vi "sq_test_all.vi"() -> ()   [LabVIEW 2012]
doc: "This VI is an example of how to use the Host VI to open the I2C bus, write, read, and close I2C bus. This VI should work for any I2C EEPROM or RAM IC. Note that many of these devices have a limit on how many bytes can be writen to the device at a time.\n\nWritten By:\nPeter Fuller\nSenior Engineer\nplf Consulting, LLC\n\nemail: peter@plfconsulting.com\nphone: 617.699.2201"
uses:
  <vilib>/Platform/TimedLoop/XDataNode/timing_clust.ctl
  <vilib>/Platform/TimedLoop/XDataNode/nitl_modes.ctl
  <vilib>/Platform/TimedLoop/XDataNode/wakeup.ctl
  <vilib>/Platform/TimedLoop/XDataNode/XDataNode.xnode
  <vilib>/Platform/TimedLoop/XDataNode/XDNodeRunTimeDep.lvlib
panel:
  in  "Send":bool
  in  "Bit rate":dbl=400000.0 min=40000.0 max=2000000.0 format="%#_3p"
  in  "Init sequences":T1={"Cluster"={"Cmd bytes"=[0, 99, 145], "Send"=FALSE}, "Cluster 2"={"Cmd bytes"=[0, 107, 145, 119, 255], "Send"=FALSE}, "Cluster 3"={"Cmd bytes"=[0, 103, 145, 119, 255], "Send"=FALSE}} {"Cluster 3"."Cmd bytes" format="%.0x"; "Cluster 2"."Cmd bytes" format="%.0x"; "Cluster"."Cmd bytes" format="%.0x"}
  in  "Cont":bool
  out "Run":bool
  in  "Steps":i32=10
  in  "Pulse count":cluster{"Pulse count 2":i16, "Array":bool[]}[](array[cluster])=[{"Pulse count 2"=0, "Array"=[FALSE, FALSE, FALSE, FALSE, FALSE, FALSE]}, {"Pulse count 2"=0, "Array"=[FALSE, FALSE, FALSE, FALSE, FALSE, FALSE]}, {"Pulse count 2"=0, "Array"=[FALSE, FALSE, FALSE, FALSE, FALSE, FALSE]}] {"Pulse count 2" min=-2047 max=2047 scale=-100.0..100.0}
  in  "Step":bool
  in  "Stop":bool
  # "Start address"
  # "First data byte"
  # "No-cal"
  # "Sweep"
  # "Incremental"
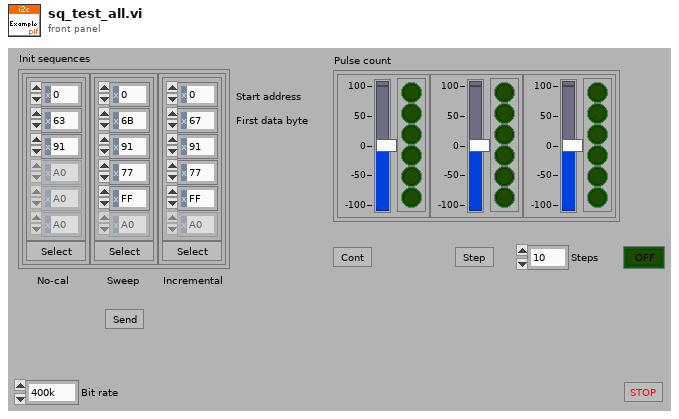
[diagram p1: front panel]
types:
  T1 = cluster{"Cluster":cluster{"Cmd bytes":u8[], "Send":bool}, "Cluster 2":cluster{"Cmd bytes":u8[], "Send":bool}, "Cluster 3":cluster{"Cmd bytes":u8[], "Send":bool}}
  T2 = typedef "i2c_interface.ctl" = cluster{"FPGA VI Reference":T3}
  T3 = typedef "fpga_reference.ctl" = refnum<k20>
  T4 = typedef "XDNodeRunTimeDep.lvlib/timing_clust.ctl" = cluster{"Expected End [f-1]":u64, "Actual End [f-1]":u64, "Finished Late? [f-1]":bool, "Expected End [i-1]":u64, "Actual End [i-1]":u64, "Finished Late? [i-1]":bool, "Expected Start [i]":u64, "Actual Start [i]":u64, "Expected Start [f]":u64, "Actual Start [f]":u64, "Source Name":string, "Structure Name":string, "Period":i64, "Deadline":i64, "Offset":i64, "Start":i64, "Priority":i32, "Timeout":i32, "Mode":T5, "Wakeup Reason":T6, "Error":errorcluster, "Source Type":string, "Secondary Source Type":string, "Global End Time":u64, "Global Start Time":u64, "Frame Duration":u64, "Iteration Duration":u64, "Assigned CPU":i32, "I/O Scan Engine Mode":u32}
  T5 = typedef "XDNodeRunTimeDep.lvlib/nitl_modes.ctl" = enum32{"No Change", "Process missed periods, maintain original phase", "Discard missed periods, maintain original phase", "Process missed periods, ignore original phase", "Discard missed periods, ignore original phase"}
  T6 = typedef "XDNodeRunTimeDep.lvlib/wakeup.ctl" = enum32{"Normal", "Aborted", "Asynchronous wakeup", "Timing source error", "Timed loop error", "Timeout"}
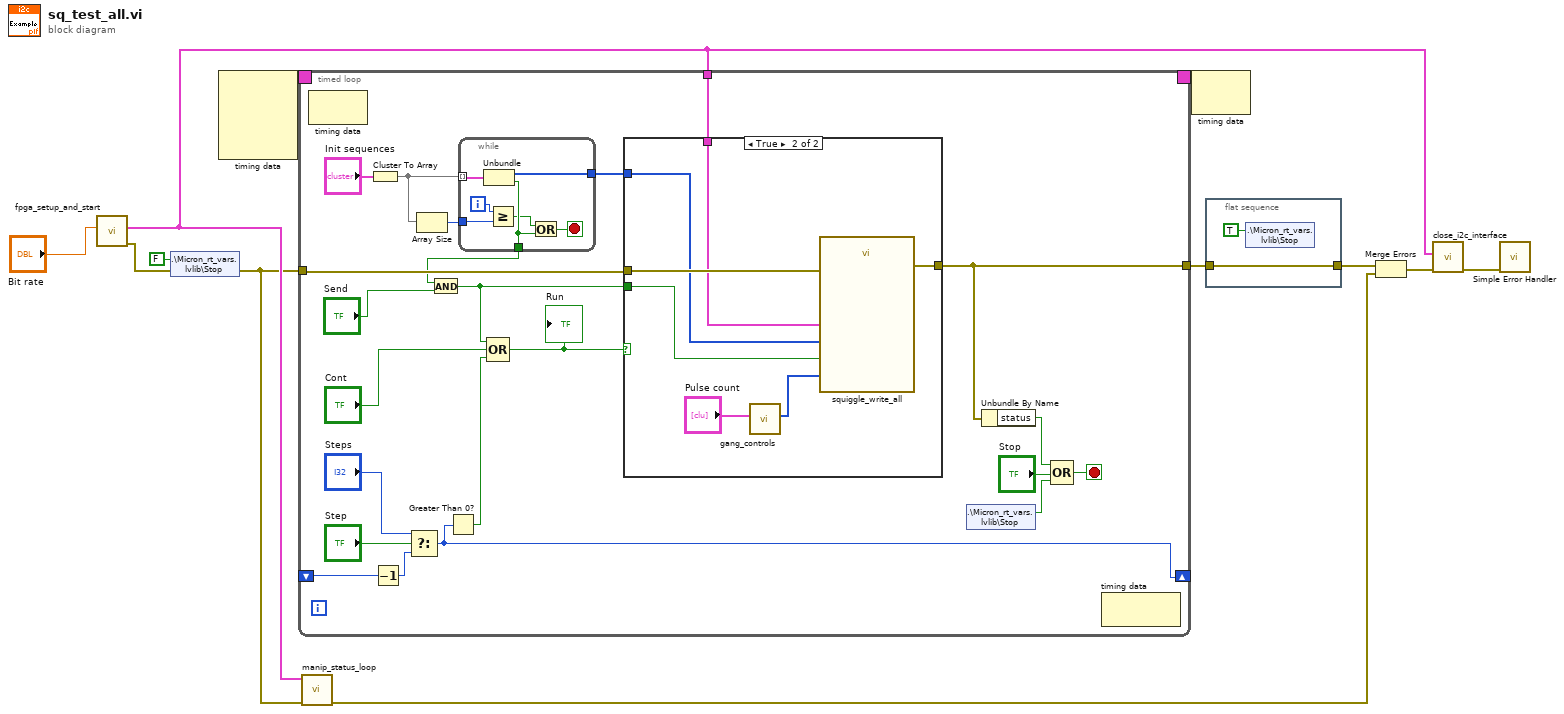
[diagram p0: block diagram]
diagram:
  n1 = call "fpga_setup_and_start.vi"("Bit rate"="Bit rate") -> ("error out"=w4:errorcluster, "I2C interface"=w8:T2)  [unwired: 9 in]
  n2 = shared-variable ".\\Micron_rt_vars.lvlib\\Stop"(FALSE ("Stop"), error in=w4) -> (error out=w3:errorcluster)
  n3 = node-c288() -> (w11:T4)  [unwired: 4 in]
  n4 = timed-loop {
    timing: w11 -> [_]
    timing-out: [_] -> w10
    tunnel: w3 -> [w34]
    tunnel: [w31] -> w1
    shift-right: [w25] -> _
    shift-left: _ -> [w26]
    tunnel: w8 -> [w18]
    stop <- w14 stop-if-true
    n5 = node-c288() -> ()  [unwired: 1 in, 1 out]
    n6 = Cluster To Array(cluster="Init sequences") -> (array=w20:cluster{"Cmd bytes":u8[], "Send":bool}[])
    n7 = Decrement(x=w26) -> (x-1=w27:i32)
    n8 = Select(t="Steps", s="Step", f=w27) -> (s? t:f=w25:i32)
    n9 = Array Size(array=w20) -> (size(s)=w19:i32)
    n10 = Greater Than 0?(x=w25) -> (x > 0?=w23:bool)
    n11 = while {
      tunnel: w20 -> [w41] mode=indexing
      tunnel: [w40] -> w22
      tunnel: [w38] -> w17
      tunnel: w19 -> [w37]
      i -> [w36]
      stop <- w39 stop-if-true
      n12 = Unbundle(w41) -> ("Cmd bytes"=w40:u8[], "Send"=w38:bool)
      n13 = Greater Or Equal?(x=w36, y=w37) -> (x >= y?=w35:bool)
      n14 = Or(x=w35, y=w38) -> (x .or. y?=w39:bool)
    }
    n15 = And(x=w17, y="Send") -> (x .and. y?=w16:bool)
    n16 = Compound Arithmetic op=OR(w16, "Cont", w23) -> (w32:bool)
    "Run" <- w32
    n17 = case shown="True" w32 {
      tunnel: w34 -> [w42 w49]
      tunnel: [w42 w47] -> w31
      tunnel: w16 -> [_ w48]
      tunnel: w22 -> [_ w44]
      tunnel: w18 -> [_ w43]
      frame False {
      }
      frame True {
        n18 = call "gang_controls.vi"("Controls"="Pulse count") -> ("Pulse count"=w45:i16[])  [unwired: 10 in]
        n19 = call "squiggle_write_all.vi"("Init sequence"=w44, "Error in"=w49, "Pulse count"=w45, "Send init sequence"=w48, "I2C interface"=w43) -> ("Error out"=w47:errorcluster)  [unwired: 6 in]
      }
    }
    n20 = shared-variable ".\\Micron_rt_vars.lvlib\\Stop"() -> (w13:bool)  [unwired: 2 out]
    n21 = Unbundle By Name(w31) -> ("status"=w30:bool)
    n22 = Compound Arithmetic op=OR(w30, "Stop", w13) -> (w14:bool)
    n23 = node-c288() -> ()  [unwired: 1 in, 1 out]
  }
  n24 = call "manip_status_loop.vi"("error in"=w3, "I2C interface"=w8) -> ("error out"=w7:errorcluster)  [unwired: 9 in]
  n25 = node-c288(w10) -> ()  [unwired: 1 out]
  n26 = flat-sequence {
    tunnel: [w52] -> w2
    tunnel: w1 -> [w52]
    frame #0 {
      n27 = shared-variable ".\\Micron_rt_vars.lvlib\\Stop"(TRUE ("Stop")) -> ()  [unwired: 2 out]
    }
  }
  n28 = Merge Errors(w2, w7) -> (w6:errorcluster)
  n29 = call "close_i2c_interface.vi"("error in"=w6, "I2C interface"=w8) -> ("error out"=w12:errorcluster)  [unwired: 9 in]
  n30 = call <vilib>:"Simple Error Handler.vi"("error in (no error)"=w12) -> ()  [unwired: 4 in, 5 out]
